vi "rad_Update AppImage Properties.vi"(7 "Temp Folder":path, 8 "error in (no error)":errorcluster, 10 "Bitfiles Modified?":bool, 11 "AppImage Information":T1) -> (0 "error out":errorcluster)   [LabVIEW 2023]
uses:
  TypeDefs/rad_AppImage Information.ctl
  TypeDefs/rad_Application Image Properties.ctl
  TypeDefs/rad_FPGA Properties.ctl
  TypeDefs/rad_FPGA Flash Properties.ctl
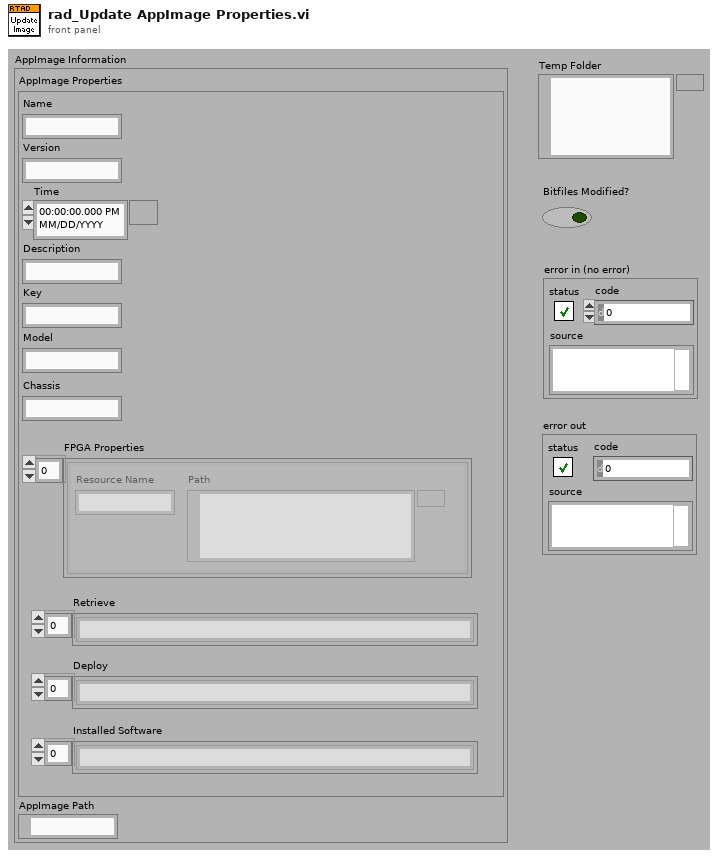
[diagram p1: front panel]
types:
  T1 = typedef "rad_AppImage Information.ctl" = cluster{"AppImage Properties":T2, "AppImage Path":path}
  T2 = typedef "rad_Application Image Properties.ctl" = cluster{"Name":string, "Version":string, "Time":timestamp, "Description":string, "Key":string, "Chassis":string, "FPGA Properties":T3, "Model":string, "Retrieve":string[], "Deploy":string[], "Installed Software":string[]}
  T3 = typedef "rad_FPGA Properties.ctl" = T4[]
  T4 = typedef "rad_FPGA Flash Properties.ctl" = cluster{"Resource Name":string, "Path":path}
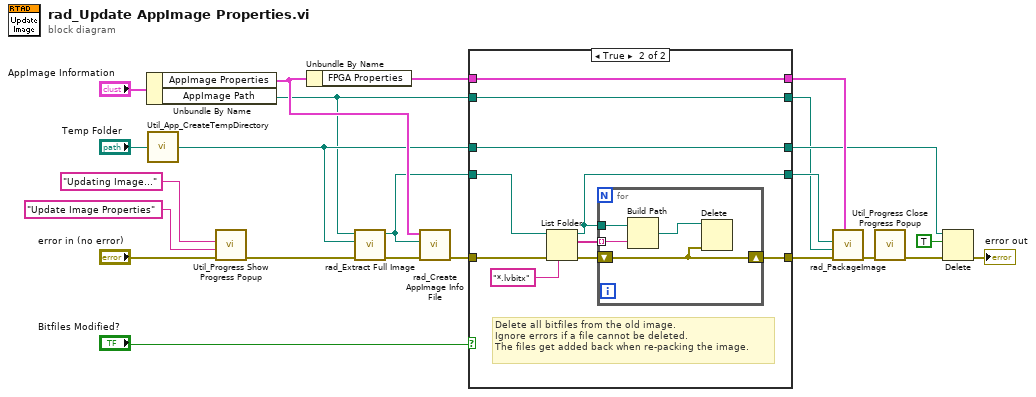
[diagram p0: block diagram]
diagram:
  n1 = Unbundle By Name("AppImage Information") -> ("AppImage Properties"=w23:T2, "AppImage Path"=w5:path)
  n2 = call "Util_App_CreateTempDirectory.vi"("TempFolderPath"="Temp Folder") -> ("TempFolderPath_out"=w8:path)
  n3 = call "Util_Progress Show Progress Popup.vi"("error in (no error)"="error in (no error)", "Title"="Update Image Properties", "Message"="Updating Image...") -> ("error out"=w2:errorcluster)  [unwired: 8 in]
  n4 = Unbundle By Name(w23) -> ("FPGA Properties"=w10:T3)
  n5 = call "rad_Extract Full Image.vi"("error in (no error)"=w2, "App Image Temp Folder"=w8, "Zipped App Image File Path"=w5) -> ("error out"=w3:errorcluster, "Unzipped App Image Folder Path"=w4:path)  [unwired: 7 in]
  n6 = call "rad_Create AppImage Info File.vi"("error in (no error)"=w3, "Temp Image Folder"=w4, "AppImage Properties"=w23) -> ("error out"=w1:errorcluster)  [unwired: 7 in, 1 out]
  n7 = case shown="True" "Bitfiles Modified?" {
    tunnel: w1 -> [w26 w37]
    tunnel: w4 -> [w24 w36]
    tunnel: [w24 w34] -> w14
    tunnel: [w26 w31] -> w12
    tunnel: w10 -> [_ w30]
    tunnel: [_ w30] -> w9
    tunnel: w8 -> [w27 w29]
    tunnel: [w27 w29] -> w7
    tunnel: w5 -> [w25 w28]
    tunnel: [w25 w28] -> w6
    frame False {
      # "Since the bitfiles did not change, do not delete\nthe old ones or add the new ones."
    }
    frame True {
      # "Delete all bitfiles from the old image.\nIgnore errors if a file cannot be deleted.\nThe files get added back when re-packing the image."
      n8 = List Folder(path=w36, pattern="*.lvbitx", error in=w37) -> (path out=w34:path, filenames=w33:string[], error out=w32:errorcluster)  [unwired: 1 in, 1 out]
      n9 = for {
        tunnel: w34 -> [w41]
        tunnel: w33 -> [w40] mode=indexing
        shift-right: [w38] -> w31
        shift-left: w32 -> [w38]
        n10 = Build Path(base path=w41, name or relative path=w40) -> (appended path=w39:path)
        n11 = Delete(path (use dialog)=w39, error in=w38) -> ()  [unwired: 3 in, 3 out]
      }
    }
  }
  n12 = call "rad_PackageImage.vi"("AppImage Properties.FPGA Properties"=w9, "error in (no error)"=w12, "AppImage Path"=w6, "Temp Image Path"=w14) -> ("error out"=w13:errorcluster)  [unwired: 7 in]
  n13 = call "Util_Progress Close Progress Popup.vi"("error in (no error)"=w13) -> ("error out"=w20:errorcluster)  [unwired: 10 in]
  n14 = Delete(path (use dialog)=w7, entire hierarchy (F)=TRUE, error in=w20) -> (error out=→"error out":errorcluster)  [unwired: 2 in, 2 out]
